vi "round 1 ques 1.vi"() -> ()   [LabVIEW 2015]
panel:
  in  "Combo Box":string(combo)
  out "Numeric":dbl
  in  "n 2":dbl
  in  "n1":dbl
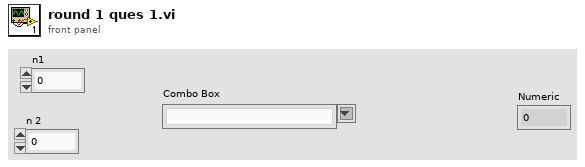
[diagram p1: front panel]
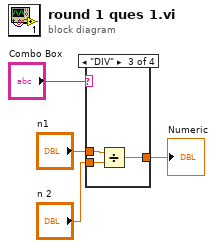
[diagram p0: block diagram]
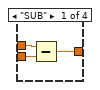
[diagram p2: hidden frame]
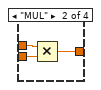
[diagram p3: hidden frame]
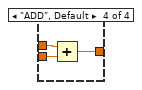
[diagram p4: hidden frame]
diagram:
  n1 = case shown="\"DIV\"" "Combo Box" {
    tunnel: "n 2" -> [w7 w10 w11 w16]
    tunnel: "n1" -> [w6 w9 w13 w15]
    tunnel: [w5 w8 w12 w14] -> w1
    frame "SUB" {
      n2 = Subtract(x=w6, y=w7) -> (x-y=w5:dbl)
    }
    frame "MUL" {
      n3 = Multiply(x=w9, y=w10) -> (x*y=w8:dbl)
    }
    frame "DIV" {
      n4 = Divide(x=w13, y=w11) -> (x/y=w12:dbl)
    }
    frame "ADD", Default {
      n5 = Add(x=w15, y=w16) -> (x+y=w14:dbl)
    }
  }
  "Numeric" <- w1
